vi "Command Turn to Cube.vi"(9 "Timeout":u32=2, 11 "Startup":bool) -> (1 "Right Wheel Velocity":dbl, 2 "Left Wheel Velocity":dbl, 3 "Reint":bool, 4 "Completed":bool=TRUE)   [LabVIEW 2017]
uses:
  Command Execution State.ctl
  Robot Global Data.vi
  Autonomous Globals.vi
panel:
  in  "Number of Checks":i32=3
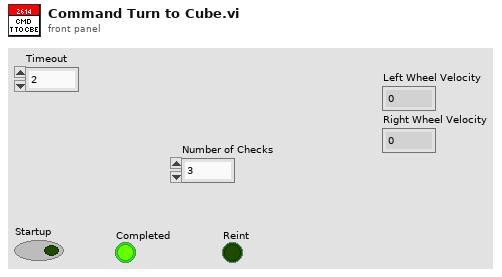
[diagram p1: front panel]
types:
  T1 = typedef "Command Execution State.ctl" = enum16{"Initialize", "Execute", "Finish"}
  T2 = cluster{"offsetAngle H":dbl, "offsetAngle V":dbl, "area":dbl, "skew":dbl}
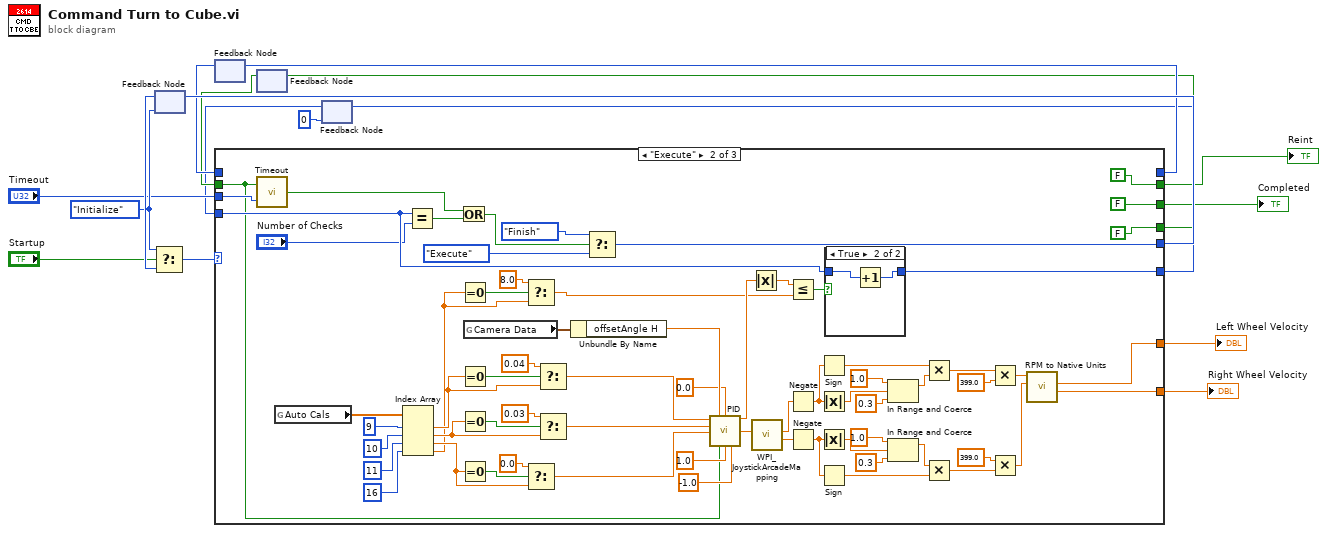
[diagram p0: block diagram]
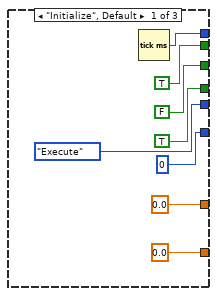
[diagram p2: hidden frame]
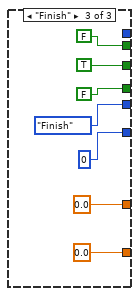
[diagram p4: hidden frame]
diagram:
  w12 = Command_Execution_State."Initialize" ("Play State")
  n1 = feedback #1(w12) -> (w15:T1)
  n2 = Select(t=w12, s="Startup", f=w15) -> (s? t:f=w17:T1)
  n3 = feedback #2() -> (w13:u32)  [unwired: 1 in]
  n4 = feedback #3() -> (w4:bool)  [unwired: 1 in]
  n5 = feedback #4(0) -> (w2:i32)
  n6 = case shown="\"Execute\"" w17 {
    tunnel: [Command_Execution_State."Execute" ("Play State") w88 Command_Execution_State."Finish" ("Play State")] -> w16
    tunnel: [w25 _ _] -> w14
    tunnel: w13 -> [_ _ _]
    tunnel: [FALSE FALSE TRUE] -> w11
    tunnel: [TRUE FALSE FALSE] -> w9
    tunnel: [0.0 w53 0.0] -> w8
    tunnel: [0.0 w54 0.0] -> w7
    tunnel: "Timeout" -> [_ w74 _]
    tunnel: [TRUE FALSE FALSE] -> w5
    tunnel: w4 -> [_ w26 _]
    tunnel: [0 w51 0] -> w3
    tunnel: w2 -> [_ w49 _]
    frame "Initialize", Default {
      n7 = Tick Count (ms)() -> (millisecond timer value=w25:u32)
    }
    frame "Execute" {
      n8 = call "Timeout.vi"("Timeout"=w74, "Initialize"=w26) -> ("Timed Out?"=w71:bool)
      n9 = global read "Autonomous Globals.vi" "Auto Cals"() -> (w47:dbl[])
      n10 = Index Array(array=w47, index #1=9 ("index"), index #2=10 ("index"), index #3=11 ("index"), index #4=16 ("index")) -> (element #1=w42:dbl, element #2=w37:dbl, element #3=w33:dbl, element #4=w27:dbl)
      n11 = Equal?(x=w49, y="Number of Checks") -> (x = y?=w50:bool)
      n12 = Or(x=w71, y=w50) -> (x .or. y?=w72:bool)
      n13 = Equal To 0?(x=w27) -> (x = 0?=w30:bool)
      n14 = Equal To 0?(x=w42) -> (x = 0?=w43:bool)
      n15 = Equal To 0?(x=w37) -> (x = 0?=w38:bool)
      n16 = Equal To 0?(x=w33) -> (x = 0?=w35:bool)
      n17 = global read "Robot Global Data.vi" "Camera Data"() -> (w86:T2)
      n18 = Select(t=8.0, s=w30, f=w27) -> (s? t:f=w29:dbl)
      n19 = Select(t=0.0, s=w35, f=w33) -> (s? t:f=w32:dbl)
      n20 = Select(t=0.04, s=w43, f=w42) -> (s? t:f=w40:dbl)
      n21 = Select(t=0.03, s=w38, f=w37) -> (s? t:f=w36:dbl)
      n22 = Unbundle By Name(w86) -> ("offsetAngle H"=w85:dbl)
      n23 = Select(t=Command_Execution_State."Finish" ("Play State"), s=w72, f=Command_Execution_State."Execute") -> (s? t:f=w88:T1)
      n24 = call "PID.vi"("Kp"=w40, "Process Variable"=w85, "Goal"=0.0, "Ki"=w36, "Kd"=w32, "Reinit"=w26, "Max Ouput"=1.0, "Min Output"=-1.0) -> ("Current Error"=w80:dbl, "Command"=w79:dbl)  [unwired: 5 in, 1 out]
      n25 = Absolute Value(x=w80) -> (abs(x)=w81:dbl)
      n26 = call <vilib>:"WPI_JoystickArcadeMapping.vi"("X axis value"=w79) -> ("Right Motor Value"=w77:dbl, "Left Motor Value"=w78:dbl)  [unwired: 9 in]
      n27 = Less Or Equal?(x=w81, y=w29) -> (x <= y?=w52:bool)
      n28 = Negate(x=w78) -> (-x=w59:dbl)
      n29 = Negate(x=w77) -> (-x=w60:dbl)
      n30 = Sign(1:w59) -> (0:w68:dbl)
      n31 = Absolute Value(x=w59) -> (abs(x)=w70:dbl)
      n32 = Absolute Value(x=w60) -> (abs(x)=w69:dbl)
      n33 = Sign(1:w60) -> (0:w65:dbl)
      n34 = case shown="True" w52 {
        tunnel: [w92 w94] -> w51
        tunnel: w49 -> [w92 w93]
        frame False {
        }
        frame True {
          n35 = Increment(x=w93) -> (x+1=w94:i32)
        }
      }
      n36 = In Range and Coerce(upper limit=1.0, x=w70, lower limit=0.3) -> (coerced(x)=w67:dbl)  [unwired: 1 out]
      n37 = In Range and Coerce(upper limit=1.0, x=w69, lower limit=0.3) -> (coerced(x)=w66:dbl)  [unwired: 1 out]
      n38 = Multiply(x=w68, y=w67) -> (x*y=w58:dbl)
      n39 = Multiply(x=w66, y=w65) -> (x*y=w57:dbl)
      n40 = Multiply(x=w58, y=399.0) -> (x*y=w56:dbl)
      n41 = Multiply(x=399.0, y=w57) -> (x*y=w55:dbl)
      n42 = call "RPM to Native Units.vi"("Right RPM"=w55, "Left RPM"=w56) -> ("Right Out"=w54:dbl, "Left Out"=w53:dbl)  [unwired: 6 in, 1 out]
    }
    frame "Finish" {
    }
  }
  "Completed" <- w11
  "Reint" <- w9
  "Left Wheel Velocity" <- w8
  "Right Wheel Velocity" <- w7
  n43 = feedback-in #1(w16) -> ()
  n44 = feedback-in #2(w14) -> ()
  n45 = feedback-in #3(w5) -> ()
  n46 = feedback-in #4(w3) -> ()
